vi "Stop Core.vi"(10 "final error code":i32, 11 "Analog Writer in":refnum<class "Analog Writer.lvclass">) -> (3 "Analog Writer out":refnum<class "Analog Writer.lvclass">)   [LabVIEW 2024, in "DAQmx Actor.lvlib" / "Analog Writer.lvclass"]
doc: "<p>(<strong>Filename</strong>: <span class=\"dnl\">Actor Framework.lvlib:Actor.lvclass:Stop Core.vi</span>)</p>\n<p>Defines what the actor does before it stops. Use the <strong>final error code</strong> input to determine whether the actor shut down in response to an error.</p>\n<p>By default, this method passes the Stop message along to all <a href=\"nihelplauncher://docs/csh?context=lvcore_lvcomm_af_launch_nested_actor\">auto-stop nested actors</a>. A descendant class may override this method to define additional behavior, such as shutting down any processes the actor initiated in its override of the <a href=\"nihelplauncher://docs/csh?context=lvcore_lvcomm_af_actor_core\">Actor Core</a> method.</p>"
uses:
  Analog Writer.lvclass
  DAQmx Actor/DAQmx Actor.lvclass
  Analog Writer.lvclass/Analog Writer.ctl
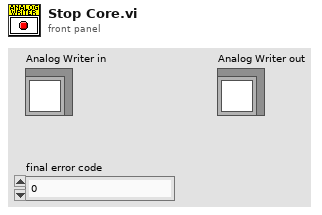
[diagram p1: front panel]
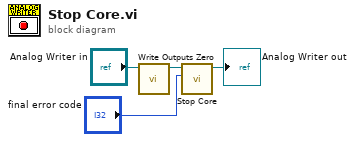
[diagram p0: block diagram]
diagram:
  n1 = call-dynamic "Write Outputs Zero.vi"("Analog Writer in"="Analog Writer in") -> ("Analog Writer out"=w1:refnum<class "Analog Writer.lvclass">)  [unwired: 9 in, 1 out]
  n2 = call-parent "Stop Core.vi"("final error code"="final error code", "DAQmx Actor in"=w1) -> ("DAQmx Actor out"=→"Analog Writer out":refnum<class "Analog Writer.lvclass">)  [unwired: 9 in]
